vi "UnMarshall.vi"(7 "Type":variant, 8 "error in (no error)":errorcluster, 10 "String":string, 11 "Serializer in":refnum<class "Serializer.lvclass">) -> (0 "error out":errorcluster, 2 "Variant":variant, 3 "Serializer out":refnum<class "Serializer.lvclass">)   [LabVIEW 2013, in "CfgManager.lvlib" / "Serializer.lvclass"]
uses:
  Serializer.lvclass
  <vilib>/Utility/VariantDataType/VariantType.lvlib
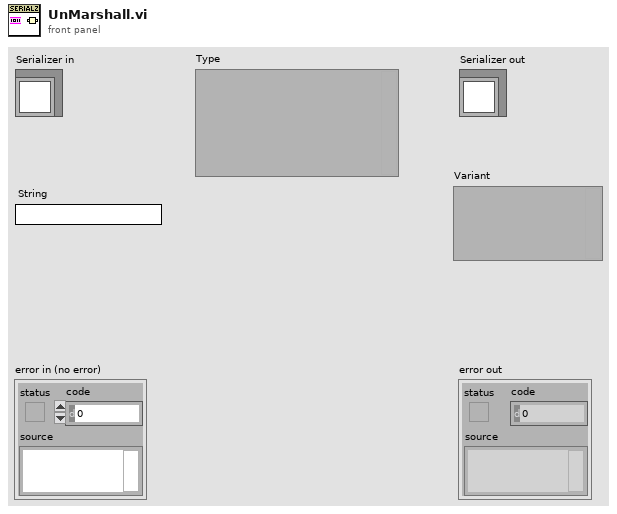
[diagram p1: front panel]
types:
  T1 = typedef "VariantType.lvlib/Type.ctl" = enum8{"Invalid Type", "Void", "I8", "I16", "I32", "I64", "U8", "U16", "U32", "U64", "Single Float", "Double Float", "Extended Float", "Single Complex", "Double Complex", "Extended Complex", "Enum U8", "Enum U16", "Enum U32", "Enum U64", "Single Float With Unit", "Double Float With Unit", "Extended Float With Unit", "Single Complex with Unit", "Double Complex with Unit", "Extended Complex with Unit", "Boolean", "String", "Path", "Picture", "Tag", "Array", "Cluster", "Variant", "LV Variant", "Waveform", "Timestamp", "Digital Waveform", "Digital Data", "ExpressData", "Refnum", "External Data", "VI", "Poly VI", "LabVIEW Class Instance", "Fixed Point"}
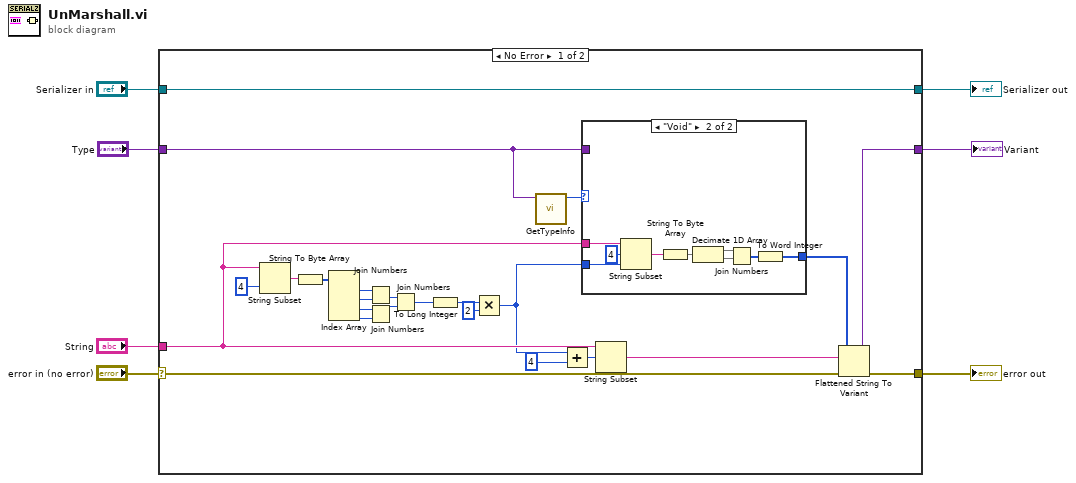
[diagram p0: block diagram]
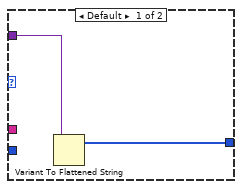
[diagram p2: hidden frame]
diagram:
  n1 = case shown="No Error" "error in (no error)" {
    selector: "error in (no error)" -> [w29 w44]
    tunnel: [w10 w44] -> w6
    tunnel: [w31 w43] -> w4
    tunnel: "Serializer in" -> [w31 w43]
    tunnel: [w27 _] -> w3
    tunnel: "Type" -> [w28 _]
    tunnel: "String" -> [w30 _]
    frame No Error {
      n2 = String Subset(string=w30, length (rest)=4 ("length (rest)")) -> (substring=w15:string)  [unwired: 1 in]
      n3 = String To Byte Array(string=w15) -> (unsigned byte array=w26:u8[])
      n4 = Index Array(array=w26) -> (element #1=w24:u8, element #2=w25:u8, element #3=w23:u8, element #4=w22:u8)  [unwired: 4 in]
      n5 = Join Numbers(hi=w24, lo=w25) -> ((hi.lo)=w20:u16)
      n6 = Join Numbers(hi=w23, lo=w22) -> ((hi.lo)=w21:u16)
      n7 = Join Numbers(hi=w20, lo=w21) -> ((hi.lo)=w9:u32)
      n8 = To Long Integer(number=w9) -> (32bit integer=w8:i32)
      n9 = Multiply(x=w8, y=2) -> (x*y=w16:i32)
      n10 = call <vilib>:"GetTypeInfo.vi"("Variant"=w28) -> ("Type Enum"=w11:T1)  [unwired: 6 in, 4 out]
      n11 = Add(x=w16, y=4 ("length (rest)")) -> (x+y=w17:i32)
      n12 = case shown="\"Void\"" w11 {
        tunnel: w30 -> [_ w42]
        tunnel: w16 -> [_ w41]
        tunnel: [w32 w34] -> w13
        tunnel: w28 -> [w33 _]
        frame Default {
          n13 = Variant To Flattened String(Variant=w33) -> (1:w32:i16[])  [unwired: 1 out]
        }
        frame "Void" {
          n14 = String Subset(string=w42, offset (0)=4 ("length (rest)"), length (rest)=w41) -> (substring=w36:string)
          n15 = String To Byte Array(string=w36) -> (unsigned byte array=w40:u8[])
          n16 = Decimate 1D Array(w40) -> (w39:u8[], w38:u8[])
          n17 = Join Numbers(hi=w39, lo=w38) -> ((hi.lo)=w37:u16[])
          n18 = To Word Integer(number=w37) -> (16bit integer=w34:i16[])
        }
      }
      n19 = String Subset(string=w30, offset (0)=w17) -> (substring=w18:string)  [unwired: 1 in]
      n20 = Flattened String To Variant(4:w29, 6:w18, 7:w13) -> (0:w10:errorcluster, 3:w27:variant)
    }
    frame Error {
    }
  }
  "error out" <- w6
  "Serializer out" <- w4
  "Variant" <- w3
